vi "select RawTestData.vi"(6 "Light > 0?":bool, 7 "Number Select":u16=10, 8 "Vmax":dbl, 9 "Vmin":dbl, 10 "V meas":dbl[](array[numeric]), 11 "I meas":dbl[](array[numeric])) -> (0 "Number Output":u32, 1 "Selected V":dbl[](array[numeric]), 2 "Selected I":dbl[](array[numeric]), 3 "Selected Index":dbl[](array[numeric]))   [LabVIEW 2012]
panel:
  out "inRange":bool[](array[boolean])
  out "index 2":u32[](array[numeric])
  out "V meas 2":dbl[](array[numeric])
  out "I meas 2":dbl[](array[numeric])
  out "index":u32[](array[numeric])
  out "sorted index":dbl[](array[numeric])
  out "sorted I":dbl[](array[numeric])
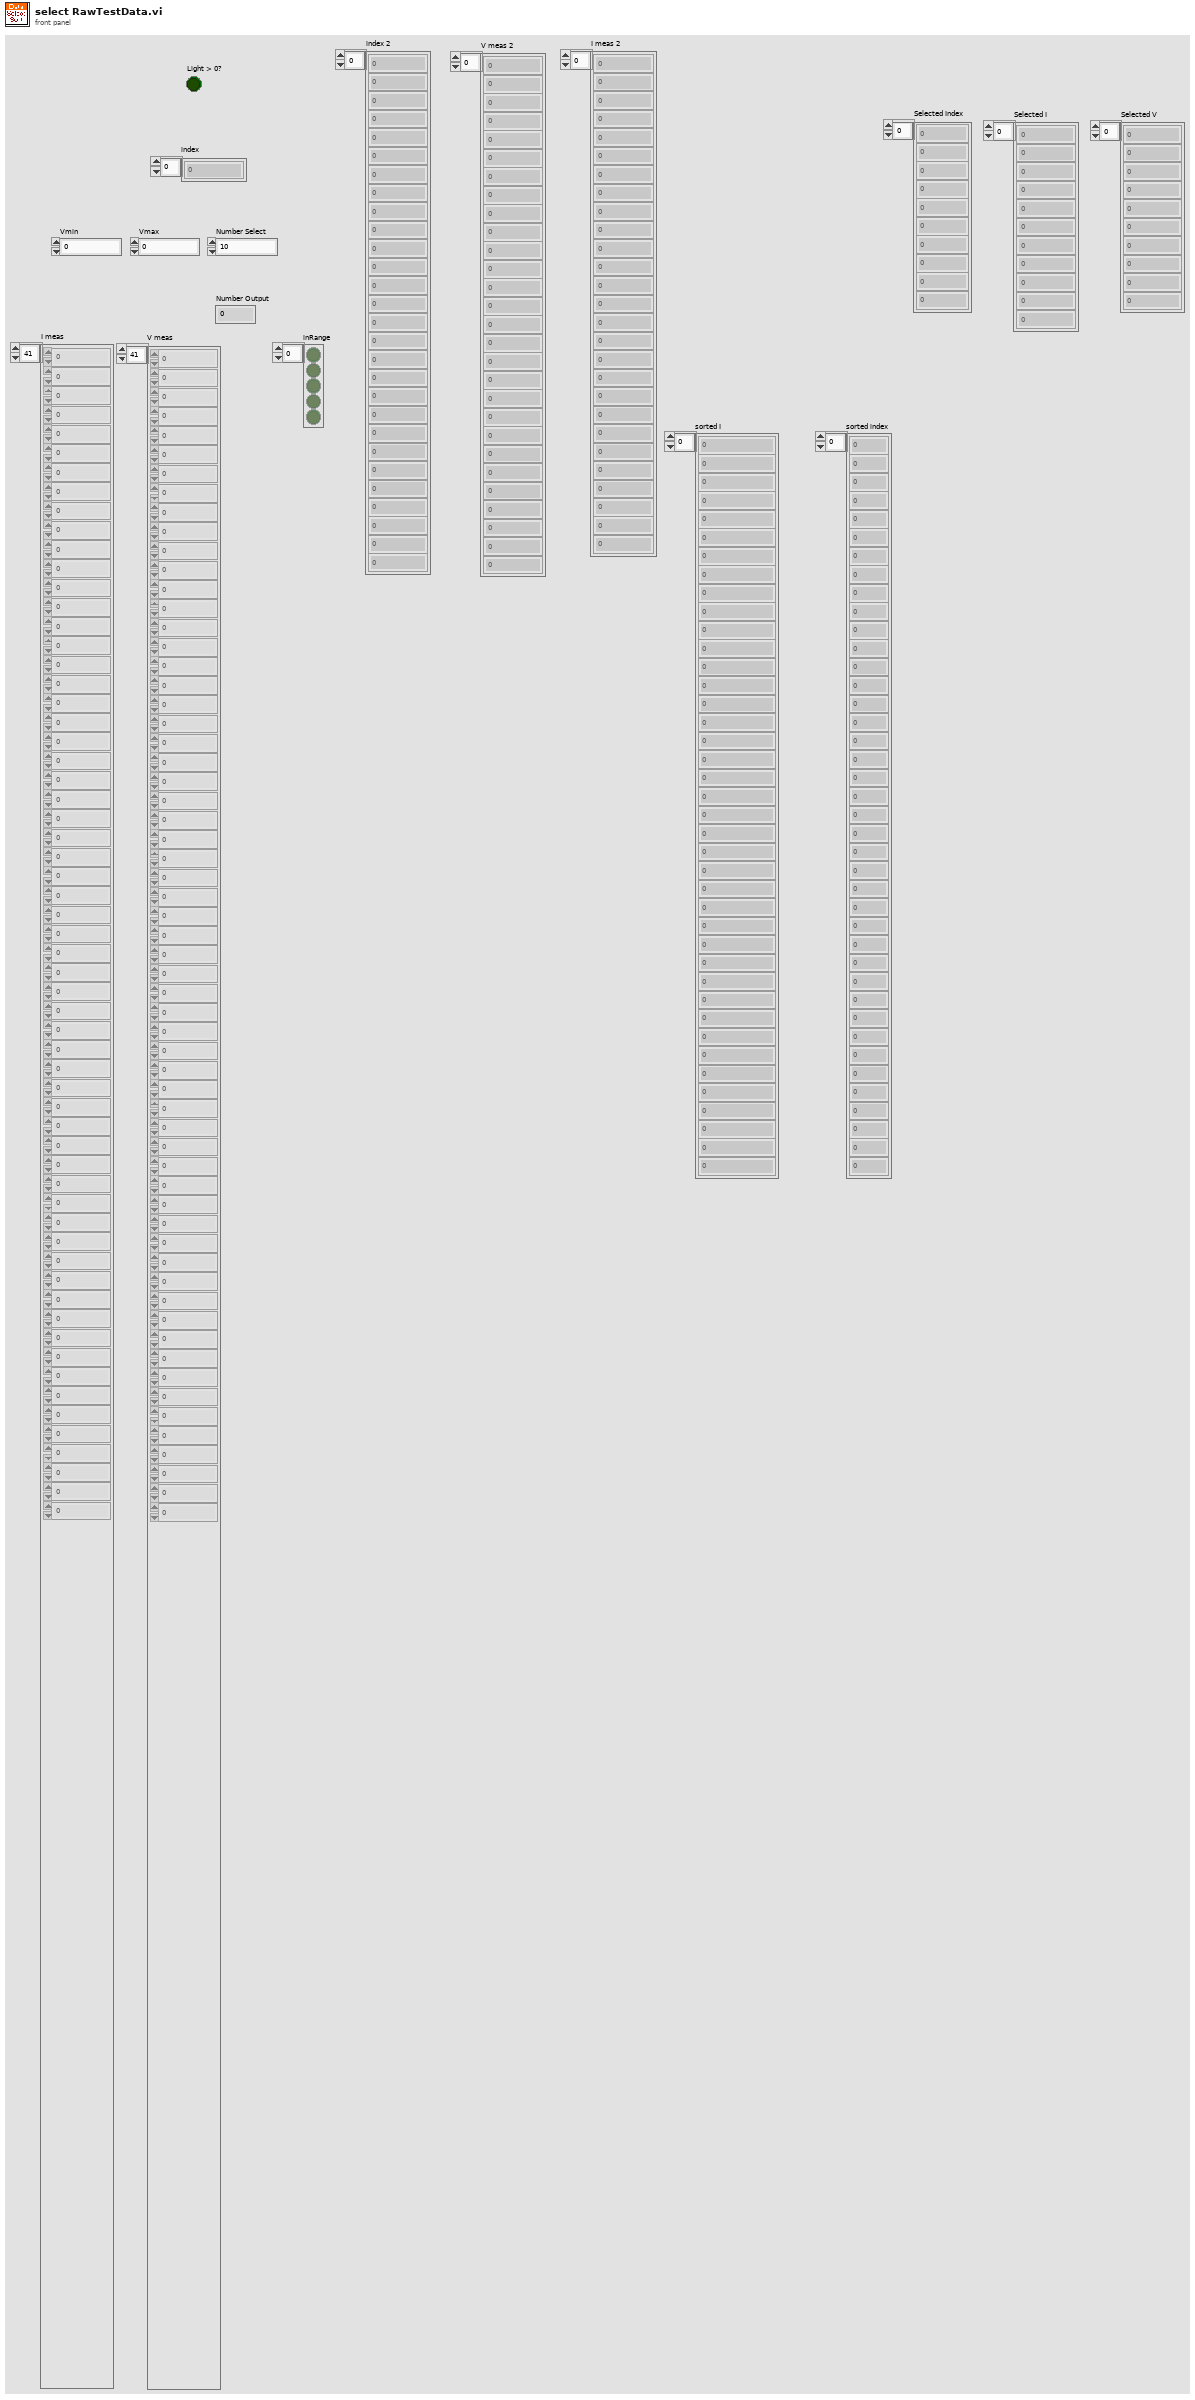
[diagram p1: front panel]
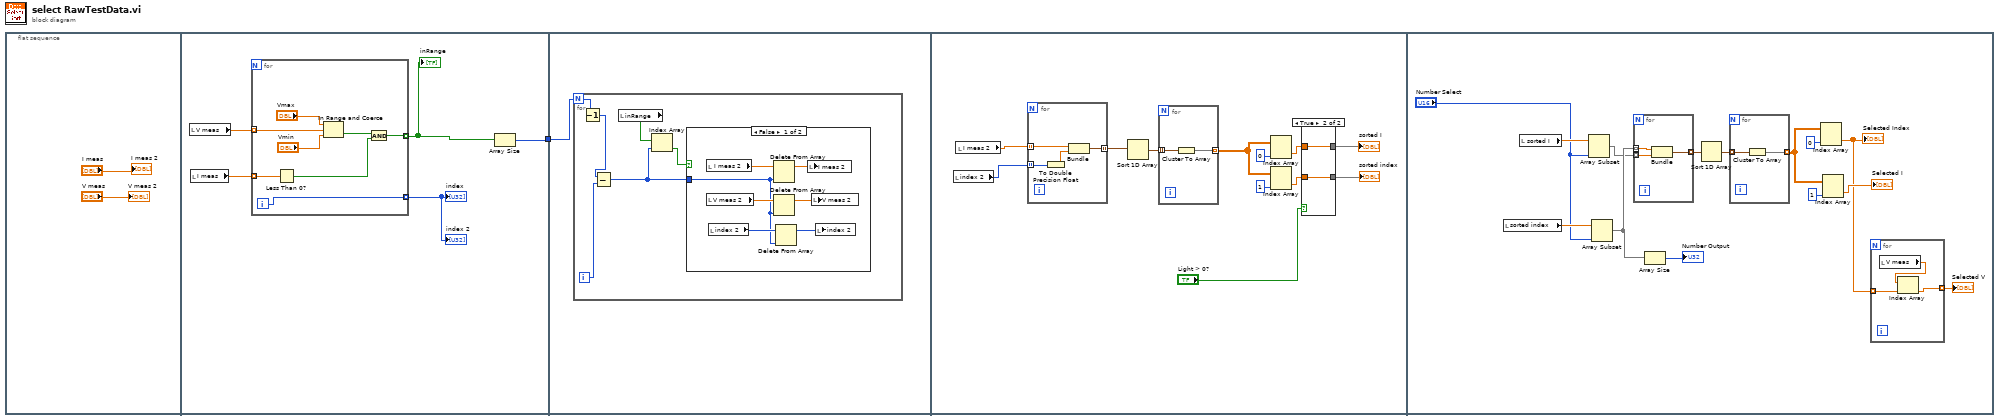
[diagram p0: block diagram]
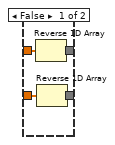
[diagram p3: hidden frame]
diagram:
  n1 = flat-sequence {
    tunnel: [w7] -> w1
    tunnel: w1 -> [w17]
    frame #0 {
      "V meas 2" <- "V meas"
      "I meas 2" <- "I meas"
    }
    frame #1 {
      n2 = local read "V meas"() -> (w6:dbl[])
      n3 = local read "I meas"() -> (w8:dbl[])
      n4 = for {
        tunnel: w6 -> [w14] mode=indexing
        tunnel: [w10] -> w4 mode=indexing
        tunnel: w8 -> [w13] mode=indexing
        tunnel: [w9] -> w5 mode=indexing
        i -> [w9]
        n5 = Less Than 0?(x=w13) -> (x < 0?=w12:bool)
        n6 = In Range and Coerce(upper limit="Vmax", x=w14, lower limit="Vmin") -> (In Range?=w11:bool)  [unwired: 1 out]
        n7 = And(x=w11, y=w12) -> (x .and. y?=w10:bool)
      }
      "index" <- w5
      "index 2" <- w5
      "inRange" <- w4
      n8 = Array Size(array=w4) -> (size(s)=w7:i32)
    }
    frame #2 {
      n9 = for {
        N: w17 -> [w19]
        i -> [w23]
        n10 = Decrement(x=w19) -> (x-1=w18:i32)
        n11 = Subtract(x=w18, y=w23) -> (x-y=w22:i32)
        n12 = local read "inRange"() -> (w20:bool[])
        n13 = Index Array(array=w20, index=w22) -> (element=w21:bool)
        n14 = case shown="False" w21 {
          tunnel: w22 -> [w24 _]
          frame False {
            n15 = local read "V meas 2"() -> (w28:dbl[])
            n16 = local read "I meas 2"() -> (w30:dbl[])
            n17 = local read "index 2"() -> (w26:u32[])
            n18 = Delete From Array(array=w30, index=w24) -> (array with subset deleted=w29:dbl[])  [unwired: 1 in, 1 out]
            n19 = Delete From Array(array=w28, index=w24) -> (array with subset deleted=w27:dbl[])  [unwired: 1 in, 1 out]
            n20 = Delete From Array(array=w26, index=w24) -> (array with subset deleted=w25:u32[])  [unwired: 1 in, 1 out]
            n21 = local write "I meas 2"(w29) -> ()
            n22 = local write "V meas 2"(w27) -> ()
            n23 = local write "index 2"(w25) -> ()
          }
          frame True {
          }
        }
      }
    }
    frame #3 {
      n24 = local read "index 2"() -> (w34:u32[])
      n25 = local read "I meas 2"() -> (w33:dbl[])
      n26 = for {
        tunnel: w33 -> [w53] mode=indexing
        tunnel: [w52] -> w42 mode=indexing
        tunnel: w34 -> [w51] mode=indexing
        n27 = To Double Precision Float(number=w51) -> (double precision float=w54:dbl)
        n28 = Bundle("Numeric"=w53, w54) -> (w52:cluster{"Numeric":dbl, dbl})  [unwired: 1 in]
      }
      n29 = Sort 1D Array(array=w42) -> (sorted array=w41:cluster{"Numeric":dbl, dbl}[])
      n30 = for {
        tunnel: w41 -> [w50] mode=indexing
        tunnel: [w49] -> w40 mode=indexing
        n31 = Cluster To Array(cluster=w50) -> (array=w49:dbl[])
      }
      n32 = Index Array(array=w40, index (col)=0 ("disabled index (col)")) -> (element=w32:dbl[])  [unwired: 1 in]
      n33 = Index Array(array=w40, index (col)=1) -> (element=w37:dbl[])  [unwired: 1 in]
      n34 = case shown="True" "Light > 0?" {
        tunnel: w37 -> [w46 w47]
        tunnel: [w45 w48] -> w36
        tunnel: [w44 w47] -> w35
        tunnel: w32 -> [w43 w48]
        frame False {
          n35 = Reverse 1D Array(array=w43) -> (reversed array=w45:dbl[])
          n36 = Reverse 1D Array(array=w46) -> (reversed array=w44:dbl[])
        }
        frame True {
        }
      }
      "sorted I" <- w36
      "sorted index" <- w35
    }
    frame #4 {
      n37 = local read "sorted index"() -> (w67:dbl[])
      n38 = local read "sorted I"() -> (w68:dbl[])
      n39 = Array Subset(array=w68, length="Number Select") -> (w59:dbl[])  [unwired: 1 in]
      n40 = Array Subset(array=w67, length="Number Select") -> (w60:dbl[])  [unwired: 1 in]
      n41 = for {
        tunnel: w60 -> [w76] mode=indexing
        tunnel: w59 -> [w75] mode=indexing
        tunnel: [w74] -> w65 mode=indexing
        n42 = Bundle("Numeric"=w76, "Numeric"=w75) -> (w74:cluster{"Numeric":dbl, "Numeric":dbl})  [unwired: 1 in]
      }
      n43 = Array Size(array=w60) -> (size(s)=→"Number Output":i32)
      n44 = Sort 1D Array(array=w65) -> (sorted array=w64:cluster{"Numeric":dbl, "Numeric":dbl}[])
      n45 = for {
        tunnel: w64 -> [w73] mode=indexing
        tunnel: [w72] -> w63 mode=indexing
        n46 = Cluster To Array(cluster=w73) -> (array=w72:dbl[])
      }
      n47 = Index Array(array=w63, index (col)=0 ("disabled index (col)")) -> (element=w57:dbl[])  [unwired: 1 in]
      "Selected Index" <- w57
      n48 = Index Array(array=w63, index (col)=1 ("disabled index (col)")) -> (element=→"Selected I":dbl[])  [unwired: 1 in]
      n49 = for {
        tunnel: w57 -> [w70] mode=indexing
        tunnel: [w69] -> w56 mode=indexing
        n50 = local read "V meas"() -> (w71:dbl[])
        n51 = Index Array(array=w71, index=w70) -> (element=w69:dbl)
      }
      "Selected V" <- w56
    }
  }
